vi "Is_TopLevel.vi"(8 "error in (no error)":errorcluster, 11 "AB_Source in":refnum<class "AB_Source.lvclass">) -> (0 "error out":errorcluster, 1 "openVIreference":bool, 2 "path":path, 3 "AB_Source out":refnum<class "AB_Source.lvclass">, 5 "readLinker":bool)   [LabVIEW 2020, in "AB_Source.lvclass"]
uses:
  <vilib>/AppBuilder/AB_Classes/Source/AB_Source.lvclass
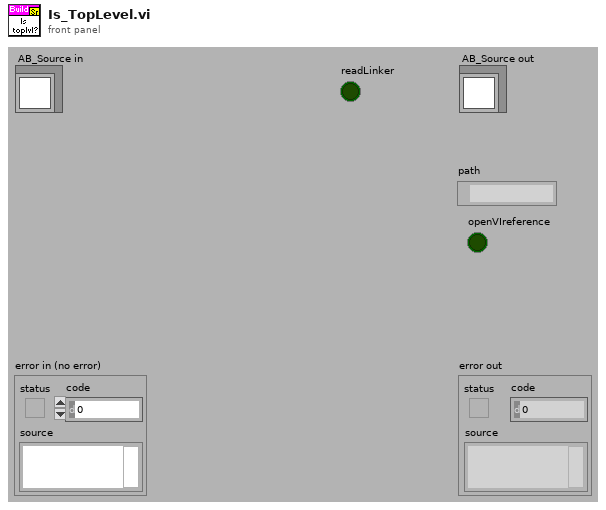
[diagram p1: front panel]
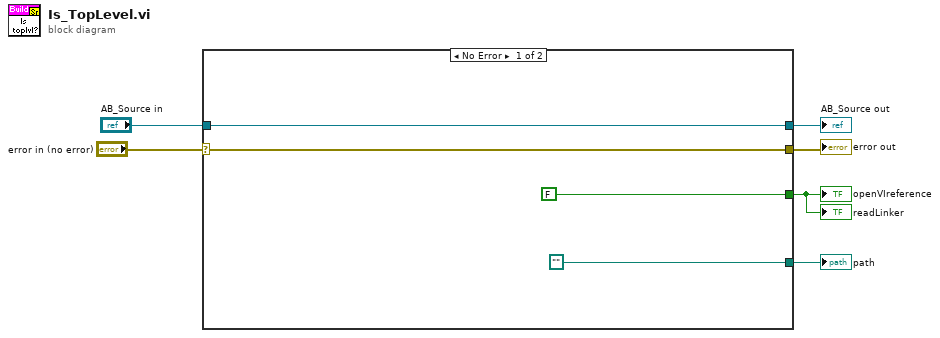
[diagram p0: block diagram]
diagram:
  n1 = case shown="No Error" "error in (no error)" {
    selector: "error in (no error)" -> [w9 w12]
    tunnel: [w9 w12] -> w5
    tunnel: [w10 w11] -> w3
    tunnel: "AB_Source in" -> [w10 w11]
    tunnel: [FALSE _] -> w1
    tunnel: [path "" _] -> w2
    frame No Error {
    }
    frame Error {
    }
  }
  "error out" <- w5
  "AB_Source out" <- w3
  "path" <- w2
  "openVIreference" <- w1
  "readLinker" <- w1
